vi "CreateProtectedEvents.vi"(8 "error in (no error)":errorcluster, 11 "SMO":refnum<class "SMO.lvclass">) -> (0 "error out":errorcluster, 3 "SMO out":refnum<class "SMO.lvclass">)   [LabVIEW 2019, in "SMO.lvclass"]
doc: "JKI State Machine Objects (SMO) 1.3.0.56\nJKI - JKI\nCopyright (c) 2017, JKI"
uses:
  SMO.lvclass
  Typedefs/StopProcessEventData--Cluster.ctl
  Typedefs/AbortProcessEventData--Cluster.ctl
  Typedefs/SMO Dependency Event--Cluster.ctl
  Typedefs/SMO Dependency Event--Enum.ctl
  SMO.lvclass/SMO.ctl
panel:
  # "For instructions on how to use the JKI State Machine Objects, examples and video tutorials, visit:\nhttp://jki.net/state-machine-objects/\n\nJKI State Machine Objects™\nhttp://jki.net/state-machine-objects/\nCopyright (C) 2005-2015, JKI <info@jki.net>\nALL RIGHTS RESERVED"
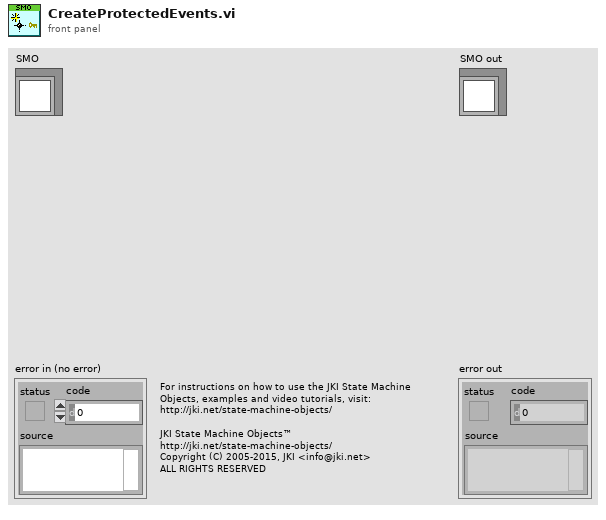
[diagram p1: front panel]
types:
  T1 = typedef "SMO.lvclass/SMO Dependency Event--Cluster.ctl" = cluster{"Name":string, "GUID":string, "Event":T2}
  T2 = typedef "SMO.lvclass/SMO Dependency Event--Enum.ctl" = enum16{"Added", "Removed", "Started", "Stopped"}
  T3 = typedef "SMO.lvclass/AbortProcessEventData--Cluster.ctl" = cluster{"Time Stamp":timestamp}
  T4 = typedef "SMO.lvclass/StopProcessEventData--Cluster.ctl" = cluster{"Time Stamp":timestamp}
  T5 = cluster{"Stop Processes":refnum<user-event>, "Abort Processes":refnum<user-event>, "Config Changed":refnum<user-event>, "Dependency Event":refnum<user-event>}
  T6 = typedef "SMO.lvclass/PrivateData--Ref.ctl" = refnum<data-value>
  T7 = typedef "SMO.lvclass/PrivateData--Cluster.ctl" = cluster{"Parent Call":T8, "Registered Processes":T9[], "Sync Notifier":refnum<notifier>, "Process Error Notifier":refnum<notifier>, "Protected Events":T10, "Public Events":T11, "SMO State":T12, "[Dependencies]":T13[], "[Attributes]":refnum<class "Attribute.lvclass">[], "Launcher Close":refnum<notifier>, "Caller Watchdog":refnum<queue>, "Accessibility":T14, "NbStaticDependencies":u32}
  T8 = typedef "SMO.lvclass/Parent Call--Enum.ctl" = enum16{"Allows parent to run", "Does not request parent to run"}
  T9 = typedef "SMO.lvclass/RegisteredProcessData--Cluster.ctl" = cluster{"Name":string, "Static VI Ref":refnum<vi>, "Running":bool, "NotifierRef":u32}
  T10 = typedef "SMO.lvclass/Protected Events.ctl" = cluster{"StopProcesses":refnum<user-event>, "AbortProcesses":refnum<user-event>, "Config Changed":refnum<user-event>, "Dependency":refnum<user-event>}
  T11 = typedef "SMO.lvclass/Public Events.ctl" = cluster{"Error":refnum<user-event>, "State":refnum<user-event>, "Reserve State":refnum<user-event>}
  T12 = typedef "SMO.lvclass/SMOState --Enum.ctl" = enum16{"unknown", "Created", "Started", "Stopped"}
  T13 = typedef "SMO.lvclass/SMO Dependency--Cluster.ctl" = cluster{"Dependency":refnum<class "SMO.lvclass">, "Level":string}
  T14 = typedef "SMO.lvclass/Accessibility--Cluster.ctl" = cluster{"Lock Key":string, "Reserve State":T15}
  T15 = typedef "SMO.lvclass/Reserve State--Enum.ctl" = enum16{"Unreserved", "Reserved", "Self-locked"}
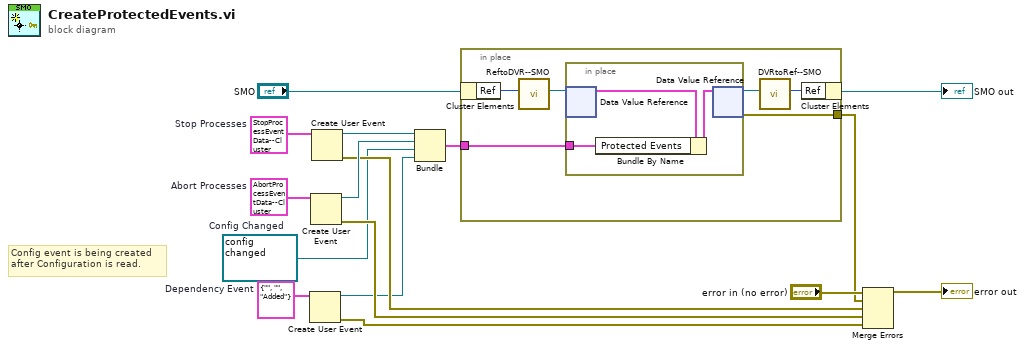
[diagram p0: block diagram]
diagram:
  w3 = T1 {"Name"="", "GUID"="", "Event"=enum."Added"}  # Dependency Event
  w4 = refnum<user-event> refnum  # Config Changed
  w10 = T3 {"Time Stamp"=timestamp(0 s since 1904-01-01)}  # Abort Processes
  w11 = T4 {"Time Stamp"=timestamp(0 s since 1904-01-01)}  # Stop Processes
  # "Config event is being created\nafter Configuration is read."
  n1 = Create User Event(user event datatype=w3) -> (user event=w2:refnum<user-event>, error out=w1:errorcluster)  [unwired: 1 in]
  n2 = Create User Event(user event datatype=w10) -> (user event=w8:refnum<user-event>, error out=w5:errorcluster)  [unwired: 1 in]
  n3 = Create User Event(user event datatype=w11) -> (user event=w9:refnum<user-event>, error out=w6:errorcluster)  [unwired: 1 in]
  n4 = Bundle("Stop Processes"=w9, "Abort Processes"=w8, "Config Changed"=w4, "Dependency Event"=w2) -> (w12:T5)  [unwired: 1 in]
  n5 = in-place {
    in-place-border: w12 -> [w22]
    in-place-border: [w21] -> w7
    n6 = in-place-cluster #1("SMO") -> ("Ref"=w20:u32)
    n7 = call "ReftoDVR--SMO.vi"("Ref"=w20) -> ("Ref"=w19:T6)  [unwired: 10 in]
    n8 = in-place {
      in-place-border: w22 -> [w23]
      n9 = in-place-dvr #2(w19) -> (w25:T7)  [unwired: 1 out]
      n10 = Bundle By Name(cluster=w25, "Protected Events"=w23) -> (w24:T7)
      n11 = in-place-dvr #2(w24) -> (w18:T6, w21:errorcluster)
    }
    n12 = call "DVRtoRef--SMO.vi"("Ref"=w18) -> ("Ref"=w17:u32)  [unwired: 10 in]
    n13 = in-place-cluster #1("Ref"=w17) -> (→"SMO out":refnum<class "SMO.lvclass">)
  }
  n14 = Merge Errors("error in (no error)", w7, w6, w5, w1) -> (→"error out":errorcluster)
